vi "try_relay.vi"(8 "Relay Status":bool, 9 "Tries":i32=5, 10 "Relay":i32=1 min=1 max=12, 11 "Slot":i32=10 min=0 max=14) -> ()   [LabVIEW 2011]
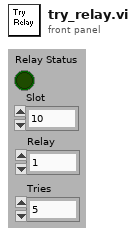
[diagram p1: front panel]
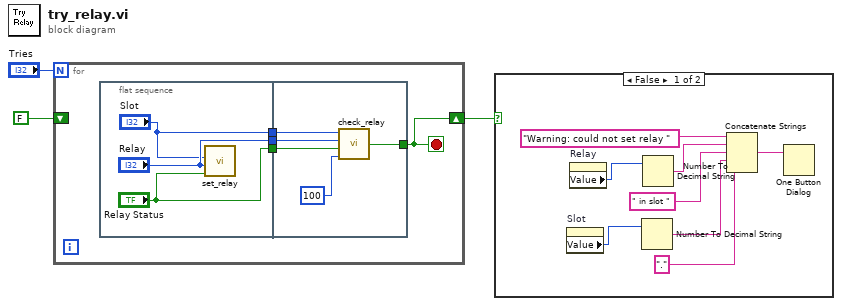
[diagram p0: block diagram]
diagram:
  n1 = for {
    N: "Tries" -> [_]
    shift-right: [w4] -> w1
    shift-left: FALSE -> [_]
    stop <- w4 stop-if-true
    n2 = flat-sequence {
      tunnel: ["Relay Status"] -> w7
      tunnel: ["Relay"] -> w6
      tunnel: ["Slot"] -> w5
      tunnel: w7 -> [w15]
      tunnel: w6 -> [w13]
      tunnel: w5 -> [w12]
      tunnel: [w11] -> w4
      frame #0 {
        n3 = call "set_relay.vi"("Slot"="Slot", "Relay"="Relay", "Relay Status"="Relay Status") -> ()  [unwired: 2 in, 1 out]
      }
      frame #1 {
        n4 = call "check_relay.vi"("Wait (ms)"=100, "Relay Status"=w15, "Relay"=w13, "Slot"=w12) -> ("success"=w11:bool)
      }
    }
  }
  n5 = case shown="False" w1 {
    frame False {
      n6 = property on="Slot" class="DigNum (strict)"() -> ("Value"=w22:i32)  [unwired: 2 in, 2 out]
      n7 = property on="Relay" class="DigNum (strict)"() -> ("Value"=w23:i32)  [unwired: 2 in, 2 out]
      n8 = Number To Decimal String(number=w22) -> (decimal integer string=w18:string)  [unwired: 1 out]
      n9 = Number To Decimal String(number=w23) -> (decimal integer string=w21:string)  [unwired: 1 out]
      n10 = Concatenate Strings("Warning: could not set relay " ("message"), w21, " in slot " ("string"), w18, "." ("string")) -> (w16:string)
      n11 = One Button Dialog(message=w16) -> ()  [unwired: 2 out]
    }
    frame True {
    }
  }
